vi "Read Serial Port Attributes.vi"(8 "error in (no error)":errorcluster, 11 "ArduinoUnoR3 in":refnum<class "ArduinoUnoR3.lvclass">) -> (0 "error out":errorcluster, 2 "Serial Port Attributes":T1={"Baud Rate"=9600, "Data Bits"=8, "Stop Bits"=10, "Data Flow"=0, "Timeout"=0, "parity (0:none)"=enum."None", "Establish Wait"=10000} {"Stop Bits" items=["1.0"=10, "1.5"=15, "2.0"=20]}, 3 "ArduinoUnoR3 out":refnum<class "ArduinoUnoR3.lvclass">)   [LabVIEW 2023, in "HAF.lvlib" / "ArduinoUnoR3.lvclass"]
doc: "Returns the attributes to use to configure the Serial Port used by this Driver."
uses:
  ArduinoUnoR3.lvclass
  ArduinoUnoR3.lvclass/ArduinoUnoR3.ctl
  SerialDriver/SerialDriver.lvclass
  Serial Port Attributes.ctl
  HAF.lvlib
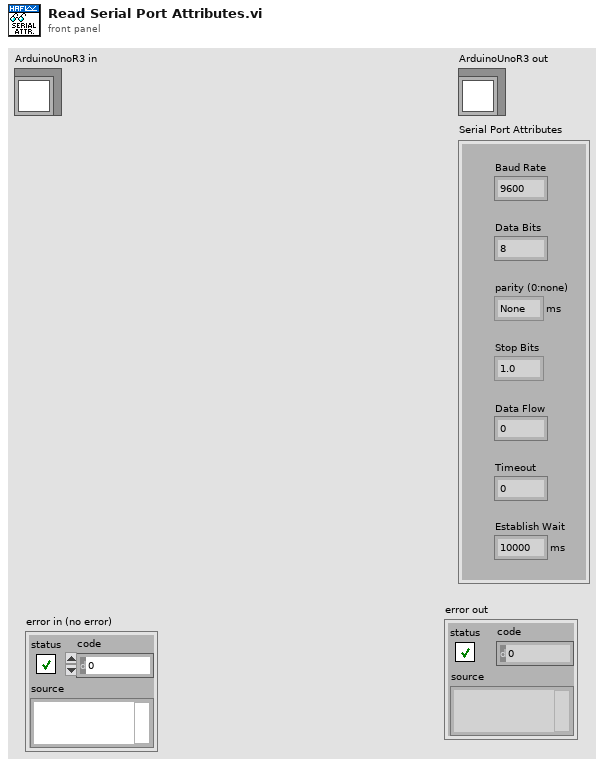
[diagram p1: front panel]
types:
  T1 = typedef "HAF.lvlib/Serial Port Attributes.ctl" = cluster{"Baud Rate":u32, "Data Bits":u16, "Stop Bits":u16, "Data Flow":u16, "Timeout":u32, "parity (0:none)":enum16{"None", "Odd", "Even", "Mark", "Space"}, "Establish Wait":u32}
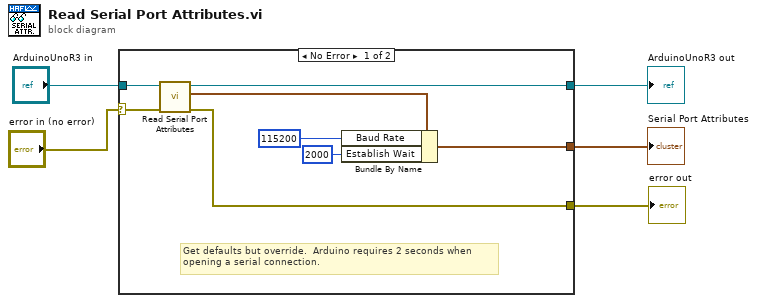
[diagram p0: block diagram]
diagram:
  n1 = case shown="No Error" "error in (no error)" {
    selector: "error in (no error)" -> [w10 w14]
    tunnel: [w13 w14] -> w5
    tunnel: [w6 _] -> w4
    tunnel: [w12 w15] -> w3
    tunnel: "ArduinoUnoR3 in" -> [w11 w15]
    frame No Error {
      # "Get defaults but override.  Arduino requires 2 seconds when\nopening a serial connection."
      n2 = call-parent "Read Serial Port Attributes.vi"("error in (no error)"=w10, "SerialDriver in"=w11) -> ("error out"=w13:errorcluster, "Serial Port Attributes"=w9:T1, "SerialDriver out"=w12:refnum<class "ArduinoUnoR3.lvclass">)  [unwired: 7 in]
      n3 = Bundle By Name(cluster=w9, "Baud Rate"=u32 115200, "Establish Wait"=u32 2000) -> (w6:T1)
    }
    frame Error {
    }
  }
  "error out" <- w5
  "ArduinoUnoR3 out" <- w3
  "Serial Port Attributes" <- w4
